vi "GetData.vi"(7 "LabVIEW Web Service Request":refnum<class "Web Request.lvclass">) -> (1 "VRMS Data":dbl, 2 "DI Data":bool[](array[boolean]), 3 "Temperature Data":dbl)   [LabVIEW 2017]
uses:
  <vilib>/wsapi/Web Request.lvclass
  Variables/GlobalData.vi
panel:
  # "Use the Web Service Request input terminal to call the VIs on the Web Services palette. Do not remove it from the connector pane unless you don't need access to the palette."
  # "Each additional control wired to the connector pane will be available as an input in the URL. To include an indicator in terminal-mode output (the default setting), it must also be wired to the connector pane."
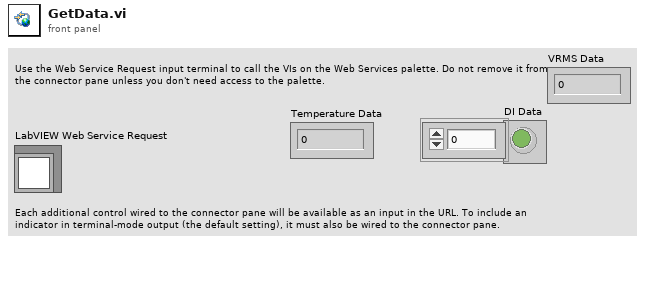
[diagram p1: front panel]
types:
  T1 = typedef "ShiftRegisterCluster.ctl" = cluster{"Temperature Task":refnum<k21>, "Temperature Data":dbl, "Encoder Task":refnum<k21>, "Encoder Data":dbl, "DI Task":refnum<k21>, "DI Data":bool[], "VRMS Task":refnum<k21>, "VRMS Data":dbl}
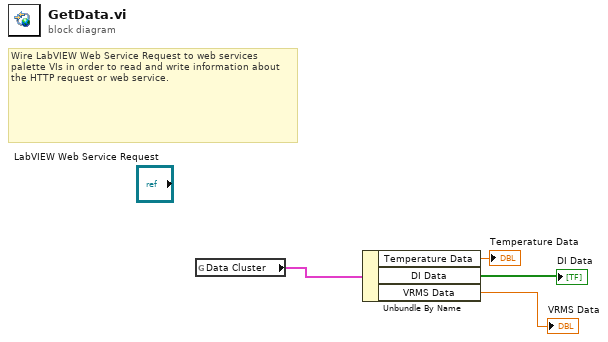
[diagram p0: block diagram]
diagram:
  # "Wire LabVIEW Web Service Request to web services palette VIs in order to read and write information about the HTTP request or web service."
  n1 = global read "GlobalData.vi" "Data Cluster"() -> (w4:T1)
  n2 = Unbundle By Name(w4) -> ("Temperature Data"=→"Temperature Data":dbl, "DI Data"=→"DI Data":bool[], "VRMS Data"=→"VRMS Data":dbl)
